vi "2019-05-07.vi"() -> ()   [LabVIEW 2018]
panel:
  out "RandomX100-50":dbl
  out "-1, 0, 1":dbl
  out "1/x":dbl
  out "-x":dbl
  out "x^2":dbl
  out "sqrt(x)":dbl
  out "x*2^n":dbl
  out "Round Toward + Infinity":dbl
  out "Round Toward - Infinity":dbl
  out "Round To Nearest Function":dbl
  out "abs(x)":dbl
  out "Random Number":dbl
  out "숫자형 8":dbl
  out "숫자형 7":dbl
  out "숫자형 6":dbl
  out "숫자형 5":dbl
  out "숫자형 4":dbl
  out "숫자형 3":dbl
  in  "숫자형 2":dbl
  in  "숫자형":dbl
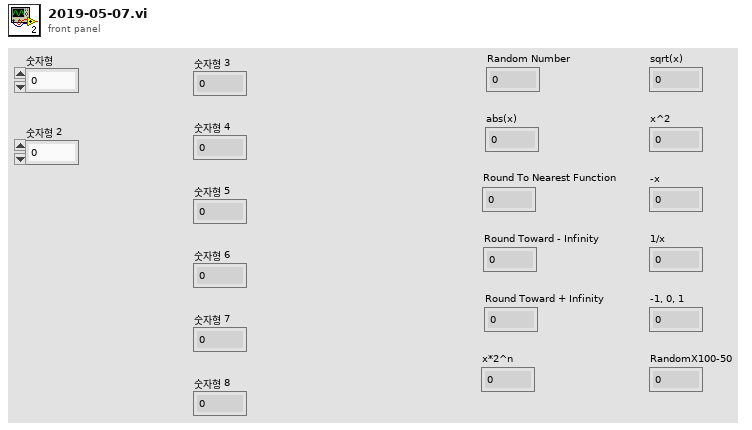
[diagram p1: front panel]
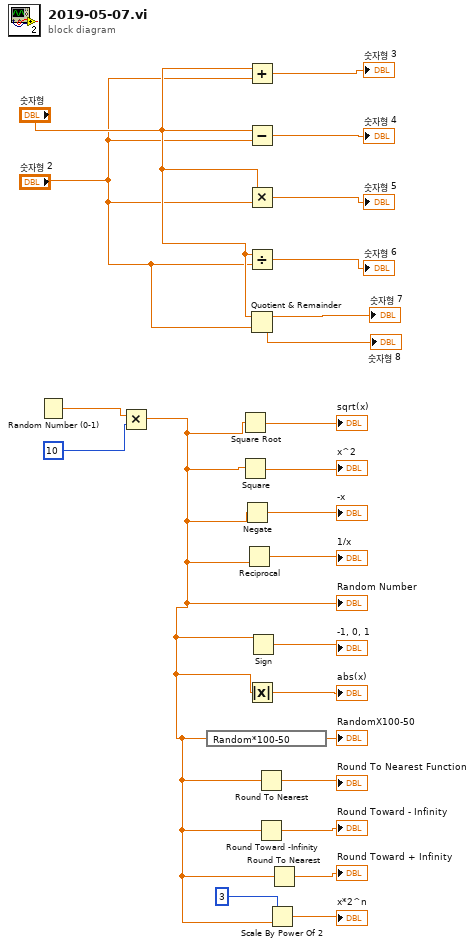
[diagram p0: block diagram]
diagram:
  n1 = Random Number (0-1)() -> (number: 0 to 1=w15:dbl)
  n2 = Multiply(x=w15, y=10) -> (x*y=w1:dbl)
  "Random Number" <- w1
  n3 = expression code="Random*100-50"(w1) -> (→"RandomX100-50":dbl)
  n4 = Square Root(x=w1) -> (sqrt(x)=→"sqrt(x)":dbl)
  n5 = Square(x=w1) -> (x^2=→"x^2":dbl)
  n6 = Negate(x=w1) -> (-x=→"-x":dbl)
  n7 = Reciprocal(x=w1) -> (1/x=→"1/x":dbl)
  n8 = Add(x="숫자형", y="숫자형 2") -> (x+y=→"숫자형 3":dbl)
  n9 = Subtract(x="숫자형", y="숫자형 2") -> (x-y=→"숫자형 4":dbl)
  n10 = Multiply(x="숫자형", y="숫자형 2") -> (x*y=→"숫자형 5":dbl)
  n11 = Divide(x="숫자형", y="숫자형 2") -> (x/y=→"숫자형 6":dbl)
  n12 = Quotient & Remainder(x="숫자형", y="숫자형 2") -> (x-y*floor(x/y)=→"숫자형 7":dbl, floor(x/y)=→"숫자형 8":dbl)
  n13 = Absolute Value(x=w1) -> (abs(x)=→"abs(x)":dbl)
  n14 = Sign(1:w1) -> (0:→"-1, 0, 1":dbl)
  n15 = Round To Nearest(number=w1) -> (nearest integer value=→"Round To Nearest Function":dbl)
  n16 = Round Toward -Infinity(1:w1) -> (0:→"Round Toward - Infinity":dbl)
  n17 = Scale By Power Of 2(n=3, x=w1) -> (x*2^n=→"x*2^n":dbl)
  n18 = Round To Nearest(number=w1) -> (nearest integer value=→"Round Toward + Infinity":dbl)
